vi "JL - Display_Blink_to_Care.vi"(7 "JL_Display_Blink":T2) -> (8 "Care?":T1)   [LabVIEW 2016]
uses:
  type defs/JL_Display_Blink.ctl
  type defs/JL Display Care.ctl
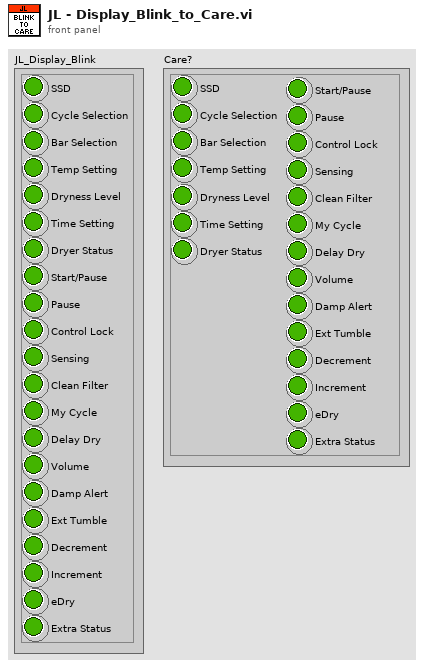
[diagram p1: front panel]
types:
  T1 = typedef "JL Display Care.ctl" = cluster{"SSD":bool, "Cycle Selection":bool, "Bar Selection":bool, "Temp Setting":bool, "Dryness Level":bool, "Time Setting":bool, "Dryer Status":bool, "Start/Pause":bool, "Pause":bool, "Control Lock":bool, "Sensing":bool, "Clean Filter":bool, "My Cycle":bool, "Delay Dry":bool, "Volume":bool, "Damp Alert":bool, "Ext Tumble":bool, "Decrement":bool, "Increment":bool, "eDry":bool, "Extra Status":bool}
  T2 = typedef "JL_Display_Blink.ctl" = cluster{"SSD":bool, "Cycle Selection":bool, "Bar Selection":bool, "Temp Setting":bool, "Dryness Level":bool, "Time Setting":bool, "Dryer Status":bool, "Start/Pause":bool, "Pause":bool, "Control Lock":bool, "Sensing":bool, "Clean Filter":bool, "My Cycle":bool, "Delay Dry":bool, "Volume":bool, "Damp Alert":bool, "Ext Tumble":bool, "Decrement":bool, "Increment":bool, "eDry":bool, "Extra Status":bool}
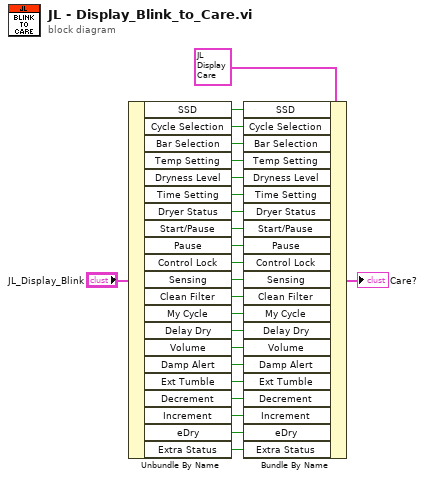
[diagram p0: block diagram]
diagram:
  n1 = Unbundle By Name("JL_Display_Blink") -> ("SSD"=w22:bool, "Cycle Selection"=w21:bool, "Bar Selection"=w20:bool, "Temp Setting"=w19:bool, "Dryness Level"=w18:bool, "Time Setting"=w17:bool, "Dryer Status"=w16:bool, "Start/Pause"=w15:bool, "Pause"=w14:bool, "Control Lock"=w13:bool, "Sensing"=w12:bool, "Clean Filter"=w11:bool, "My Cycle"=w10:bool, "Delay Dry"=w9:bool, "Volume"=w8:bool, "Damp Alert"=w7:bool, "Ext Tumble"=w6:bool, "Decrement"=w5:bool, "Increment"=w4:bool, "eDry"=w3:bool, "Extra Status"=w2:bool)
  n2 = Bundle By Name(cluster=T1 {"SSD"=FALSE, "Cycle Selection"=FALSE, "Bar Selection"=FALSE, "Temp Setting"=FALSE, "Dryness Level"=FALSE, "Time Setting"=FALSE, "Dryer Status"=FALSE, "Start/Pause"=FALSE, "Pause"=FALSE, "Control Lock"=FALSE, "Sensing"=FALSE, "Clean Filter"=FALSE, "My Cycle"=FALSE, "Delay Dry"=FALSE, "Volume"=FALSE, "Damp Alert"=FALSE, "Ext Tumble"=FALSE, "Decrement"=FALSE, "Increment"=FALSE, "eDry"=FALSE, "Extra Status"=FALSE} ("Care?"), "SSD"=w22, "Cycle Selection"=w21, "Bar Selection"=w20, "Temp Setting"=w19, "Dryness Level"=w18, "Time Setting"=w17, "Dryer Status"=w16, "Start/Pause"=w15, "Pause"=w14, "Control Lock"=w13, "Sensing"=w12, "Clean Filter"=w11, "My Cycle"=w10, "Delay Dry"=w9, "Volume"=w8, "Damp Alert"=w7, "Ext Tumble"=w6, "Decrement"=w5, "Increment"=w4, "eDry"=w3, "Extra Status"=w2) -> (→"Care?":T1)
